vi "_PC_MS manageSignalData.vi"(1 "Sig Queue":refnum<queue>, 3 "Conn_Bool":refnum<data-value>, 5 "Reload_QMH":refnum<class "QMH.lvclass">, 9 "Save_QMH":refnum<class "QMH.lvclass">, 11 "error in (no error)":errorcluster, 12 "exeObjRefnum":T1) -> ()   [LabVIEW 2018]
uses:
  PublicSubVI/Class/QMH/QMH.lvclass
  <vilib>/Utility/error.llb/Error Cluster From Error Code.vi
  <vilib>/ErrorRing/Error Ring.xnode
  PublicSubVI/Class/Sig2MS/Sig2MS.lvclass
  PublicSubVI/Class/SigInfo/SigInfo.lvclass
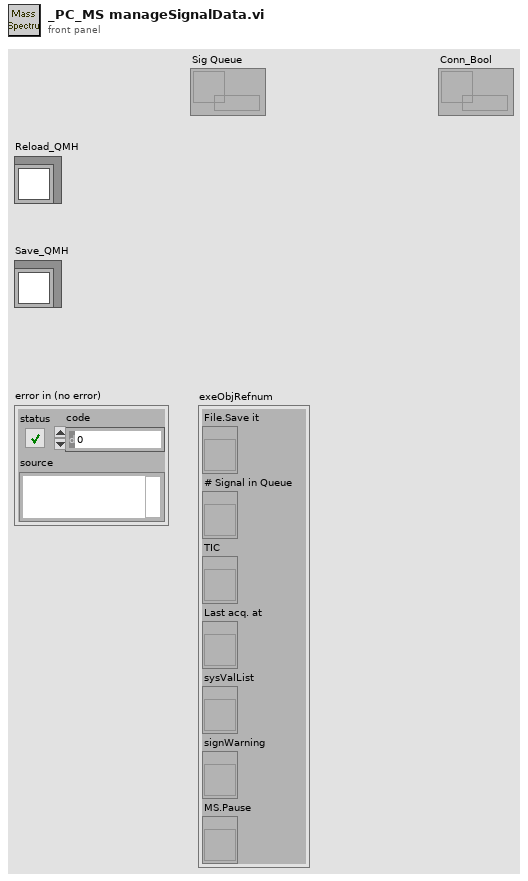
[diagram p1: front panel]
types:
  T1 = cluster{"File.Save it":refnum<vi>, "# Signal in Queue":refnum<vi>, "TIC":refnum<vi>, "Last acq. at":refnum<vi>, "sysValList":refnum<vi>, "signWarning":refnum<vi>, "MS.Pause":refnum<vi>}
  T2 = cluster{"startTime":dbl, "scanSig":cluster{"priDt":dbl, "priXData":dbl[], "priYData":sgl[], "beta":dbl[]}[], "ionSig":cluster{"secDt":dbl, "secYData":sgl[]}[]}
  T3 = enum16{"init", "loadScript", "newScript", "runScript", "close"}
  T4 = cluster{"startTime":dbl, "scanData":cluster{"dt":dbl, "xdata":dbl[], "ydata":sgl[], "beta":dbl[]}[], "xyXLabel":string, "xyYLabel":string, "wfmXLabel":string, "wfmYLabel":string, "ionData":cluster{"dt":dbl, "ydata":sgl[]}[], "ionXLabel":string, "ionYLabel":string}
  T5 = cluster{"laser_param":string, "pressure_param":cluster{"Chamber":dbl}, "turbo_param":cluster{"Speed":dbl, "Power":dbl, "rot. speed":dbl}}
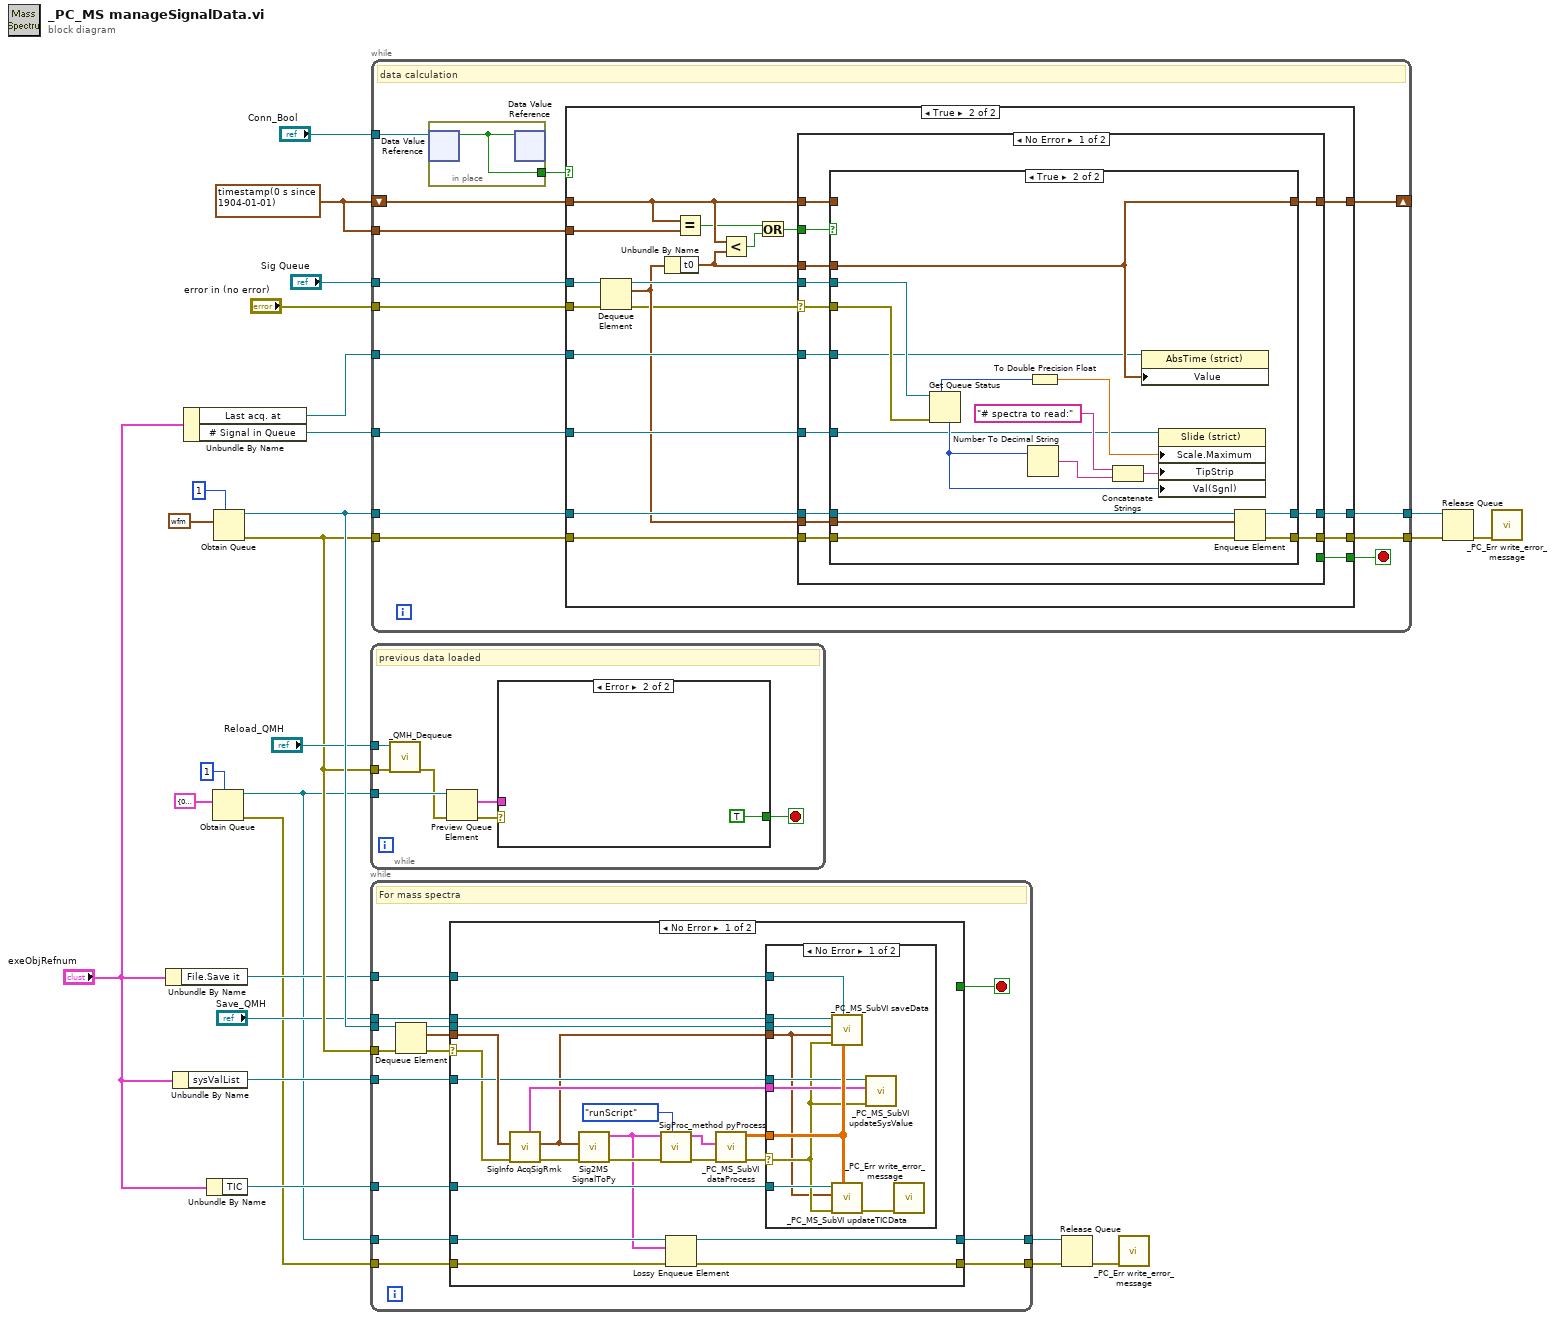
[diagram p0: block diagram]
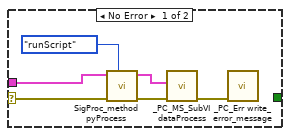
[diagram p2: hidden frame]
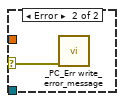
[diagram p3: hidden frame]
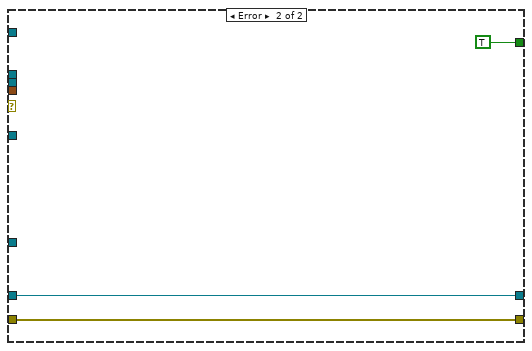
[diagram p4: hidden frame]
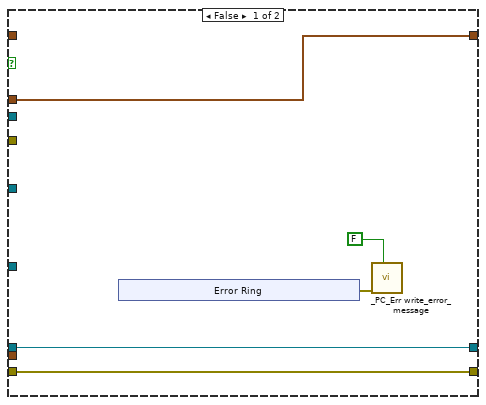
[diagram p6: hidden frame]
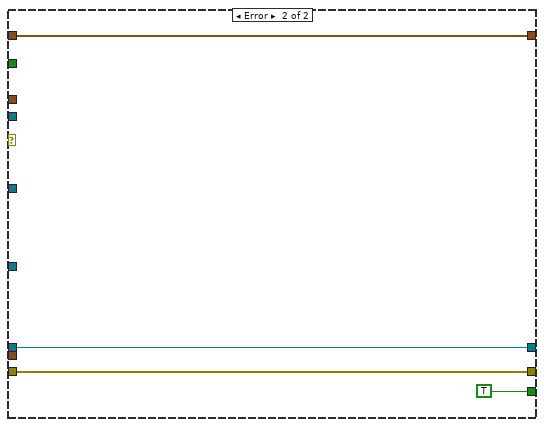
[diagram p7: hidden frame]
diagram:
  w8 = timestamp(0 s since 1904-01-01) ("t0")
  n1 = Unbundle By Name("exeObjRefnum") -> ("File.Save it"=w13:refnum<vi>)
  n2 = Unbundle By Name("exeObjRefnum") -> ("sysValList"=w11:refnum<vi>)
  n3 = Unbundle By Name("exeObjRefnum") -> ("Last acq. at"=w18:refnum<vi>, "# Signal in Queue"=w19:refnum<vi>)
  n4 = Unbundle By Name("exeObjRefnum") -> ("TIC"=w15:refnum<vi>)
  n5 = Obtain Queue(max queue size (-1, unlimited)=1, element data type=T2 {"startTime"=0.0, "scanSig"=[], "ionSig"=[]} ("pySigFormat")) -> (queue out=w7:refnum<queue>, error out=w6:errorcluster)  [unwired: 3 in, 1 out]
  n6 = Obtain Queue(max queue size (-1, unlimited)=1, element data type=waveform(sgl) {"t0"=timestamp(0 s since 1904-01-01), "dt"=1.0, "Y"=[]} ("Element out")) -> (queue out=w25:refnum<queue>, error out=w23:errorcluster)  [unwired: 3 in, 1 out]
  n7 = while {
    tunnel: "Reload_QMH" -> [w33]
    tunnel: w23 -> [w32]
    tunnel: w7 -> [w31]
    stop <- w27 stop-if-true
    # "previous data loaded"
    n8 = call "_QMH_Dequeue.vi"("error in (no error)"=w32, "QMH in"=w33) -> ("error out"=w30:errorcluster)  [unwired: 4 in, 5 out]
    n9 = Preview Queue Element(queue=w31, error in (no error)=w30) -> (element=w29:T2, error out=w28:errorcluster)  [unwired: 1 in, 2 out]
    n10 = case shown="Error" w28 {
      selector: w28 -> [w35 _]
      tunnel: w29 -> [w39 _]
      tunnel: [_ TRUE] -> w27
      frame No Error {
        n11 = call "SigProc_method pyProcess.vi"("func"=T3."runScript", "error in (no error)"=w35, "dataParam"=w39) -> ("error out"=w37:errorcluster, "newSigInfo"=w38:T4)  [unwired: 5 in, 2 out]
        n12 = call "_PC_MS_SubVI dataProcess.vi"("error in (no error)"=w37, "newSigInfo"=w38) -> ("error out"=w36:errorcluster)  [unwired: 8 in, 1 out]
        n13 = call "_PC_Err write_error_message.vi"("error in"=w36) -> ()  [unwired: 10 in, 1 out]
      }
      frame Error {
      }
    }
  }
  n14 = while {
    tunnel: w25 -> [w54]
    tunnel: w23 -> [w52]
    tunnel: w15 -> [w53]
    tunnel: "Save_QMH" -> [w47]
    tunnel: w13 -> [w50]
    tunnel: w11 -> [w48]
    tunnel: w7 -> [w45]
    tunnel: w6 -> [w44]
    tunnel: [w42] -> w5
    tunnel: [w41] -> w4
    stop <- w43 stop-if-true
    # "For mass spectra"
    n15 = Dequeue Element(queue=w54, error in (no error)=w52) -> (queue out=w51:refnum<queue>, element=w49:waveform(sgl), error out=w46:errorcluster)  [unwired: 1 in, 1 out]
    n16 = case shown="No Error" w46 {
      selector: w46 -> [w62 _]
      tunnel: w53 -> [w75 _]
      tunnel: w51 -> [w74 _]
      tunnel: w50 -> [w55 _]
      tunnel: w49 -> [w73 _]
      tunnel: w48 -> [w71 _]
      tunnel: w47 -> [w67 _]
      tunnel: w45 -> [w61 w88]
      tunnel: w44 -> [w60 w87]
      tunnel: [_ TRUE] -> w43
      tunnel: [w59 w88] -> w42
      tunnel: [w58 w87] -> w41
      frame No Error {
        n17 = call "SigInfo AcqSigRmk.vi"("error in (no error)"=w62, "signal in"=w73) -> ("error out"=w69:errorcluster, "signal out"=w70:waveform(sgl), "sys_value_param"=w72:T5)  [unwired: 7 in]
        n18 = call "Sig2MS SignalToPy.vi"("error in (no error)"=w69, "rawSignal"=w70) -> ("error out"=w68:errorcluster, "pySigFormat"=w57:T2)  [unwired: 8 in]
        n19 = call "SigProc_method pyProcess.vi"("func"=T3."runScript", "error in (no error)"=w68, "dataParam"=w57) -> ("error out"=w65:errorcluster, "newSigInfo"=w66:T4)  [unwired: 5 in, 2 out]
        n20 = Lossy Enqueue Element(queue=w61, element=w57, error in (no error)=w60) -> (queue out=w59:refnum<queue>, error out=w58:errorcluster)  [unwired: 2 out]
        n21 = call "_PC_MS_SubVI dataProcess.vi"("error in (no error)"=w65, "newSigInfo"=w66) -> ("error out"=w63:errorcluster, "ydata"=w64:sgl[][])  [unwired: 8 in]
        n22 = case shown="No Error" w63 {
          selector: w63 -> [w78 w86]
          tunnel: w67 -> [w85 _]
          tunnel: w75 -> [w84 _]
          tunnel: w74 -> [w83 _]
          tunnel: w70 -> [w77 _]
          tunnel: w64 -> [w81 _]
          tunnel: w72 -> [w80 _]
          tunnel: w71 -> [w79 _]
          tunnel: w55 -> [w76 _]
          frame No Error {
            n23 = call "_PC_MS_SubVI saveData.vi"("ydata"=w81, "File.Save it"=w76, "error in (no error)"=w78, "element"=w77, "Data Queue"=w83, "Save_QMH"=w85) -> ()  [unwired: 6 in]
            n24 = call "_PC_MS_SubVI updateTICData.vi"("ydata"=w81, "error in (no error)"=w78, "element"=w77, "TIC Graph"=w84) -> ("error out"=w82:errorcluster)  [unwired: 7 in]
            n25 = call "_PC_MS_SubVI updateSysValue.vi"("error in (no error)"=w78, "sys_value_param"=w80, "sys_value_list"=w79) -> ()  [unwired: 8 in, 1 out]
            n26 = call "_PC_Err write_error_message.vi"("error in"=w82) -> ()  [unwired: 10 in, 1 out]
          }
          frame Error {
            n27 = call "_PC_Err write_error_message.vi"("error in"=w86) -> ()  [unwired: 10 in, 1 out]
          }
        }
      }
      frame Error {
      }
    }
  }
  n28 = while {
    tunnel: "Sig Queue" -> [w103]
    tunnel: w23 -> [w98]
    tunnel: w25 -> [w99]
    tunnel: "error in (no error)" -> [w102]
    tunnel: w19 -> [w101]
    tunnel: w18 -> [w100]
    shift-right: [w97] -> _
    shift-left: w8 -> [w96]
    tunnel: "Conn_Bool" -> [w95]
    tunnel: [w93] -> w10
    tunnel: [w92] -> w9
    tunnel: w8 -> [w91]
    stop <- w90 stop-if-true
    # "data calculation"
    n29 = in-place {
      in-place-border: [w104] -> w94
      n30 = in-place-dvr #1(w95) -> (w104:bool)  [unwired: 1 out]
      n31 = in-place-dvr #1(w104) -> ()  [unwired: 2 out]
    }
    n32 = case shown="True" w94 {
      tunnel: w103 -> [_ w126]
      tunnel: w102 -> [_ w125]
      tunnel: w101 -> [_ w124]
      tunnel: w100 -> [_ w122]
      tunnel: w99 -> [w106 w121]
      tunnel: w98 -> [w105 w120]
      tunnel: [w107 w119] -> w97
      tunnel: w96 -> [w107 w116]
      tunnel: [w106 w112] -> w93
      tunnel: [w105 w111] -> w92
      tunnel: w91 -> [_ w109]
      tunnel: [_ w108] -> w90
      frame False {
      }
      frame True {
        n33 = Dequeue Element(queue=w126, error in (no error)=w125) -> (queue out=w123:refnum<queue>, element=w118:waveform(sgl), error out=w110:errorcluster)  [unwired: 1 in, 1 out]
        n34 = Unbundle By Name(w118) -> ("t0"=w117:timestamp)
        n35 = Equal?(x=w116, y=w109) -> (x = y?=w115:bool)
        n36 = Less?(x=w116, y=w117) -> (x < y?=w114:bool)
        n37 = Or(x=w115, y=w114) -> (x .or. y?=w113:bool)
        n38 = case shown="No Error" w110 {
          selector: w110 -> [w127 _]
          tunnel: w124 -> [w139 _]
          tunnel: w123 -> [w138 _]
          tunnel: w122 -> [w137 _]
          tunnel: w121 -> [w136 w168]
          tunnel: w120 -> [w135 w167]
          tunnel: [w134 w166] -> w119
          tunnel: w118 -> [w133 _]
          tunnel: w117 -> [w132 _]
          tunnel: w116 -> [w131 w166]
          tunnel: w113 -> [w130 _]
          tunnel: [w129 w168] -> w112
          tunnel: [w128 w167] -> w111
          tunnel: [_ TRUE] -> w108
          frame No Error {
            n39 = case shown="True" w130 {
              tunnel: w139 -> [_ w152]
              tunnel: w138 -> [_ w164]
              tunnel: w137 -> [_ w153]
              tunnel: w136 -> [w141 w163]
              tunnel: w135 -> [w140 w162]
              tunnel: w127 -> [_ w155]
              tunnel: [w143 w154] -> w134
              tunnel: w133 -> [_ w151]
              tunnel: w131 -> [_ _]
              tunnel: w132 -> [w143 w154]
              tunnel: [w141 w150] -> w129
              tunnel: [w140 w149] -> w128
              frame False {
                n40 = xnode "Error Ring"() -> ("error out"=w144:errorcluster)
                n41 = call "_PC_Err write_error_message.vi"("show msg( T )"=FALSE, "error in"=w144) -> ()  [unwired: 9 in, 1 out]
              }
              frame True {
                n42 = Get Queue Status(queue=w164, error in (no error)=w155) -> (max queue size=w158:i32, # elements in queue=w157:i32)  [unwired: 1 in, 6 out]
                n43 = Number To Decimal String(number=w157) -> (decimal integer string=w159:string)  [unwired: 1 in]
                n44 = To Double Precision Float(number=w158) -> (double precision float=w156:dbl)
                n45 = Concatenate Strings("# spectra to read:", w159) -> (w161:string)
                n46 = property class="AbsTime (strict)"(reference=w153, "Value"=w154) -> ()  [unwired: 1 in, 2 out]
                n47 = property class="Slide (strict)"(reference=w152, "Scale.Maximum"=w156, "TipStrip"=w161, "Val(Sgnl)"=w157) -> ()  [unwired: 1 in, 2 out]
                n48 = Enqueue Element(queue=w163, element=w151, error in (no error)=w162) -> (queue out=w150:refnum<queue>, error out=w149:errorcluster)  [unwired: 1 in, 1 out]
              }
            }
          }
          frame Error {
          }
        }
      }
    }
  }
  n49 = Release Queue(queue=w5, error in (no error)=w4) -> (error out=w2:errorcluster)  [unwired: 1 in, 2 out]
  n50 = call "_PC_Err write_error_message.vi"("error in"=w2) -> ()  [unwired: 10 in, 1 out]
  n51 = Release Queue(queue=w10, error in (no error)=w9) -> (error out=w3:errorcluster)  [unwired: 1 in, 2 out]
  n52 = call "_PC_Err write_error_message.vi"("error in"=w3) -> ()  [unwired: 10 in, 1 out]
